vi "Tegam4040 -- Test Set-GetFilterMode.vi"() -> ()   [LabVIEW 2010]
panel:
  out "LP Filter Get":enum16{"No Filter", "100kHz", "1MHz"}(ring)
  in  "LP Filter Set":enum16{"No Filter", "100kHz", "1MHz"}(ring)
  out "error out":errorcluster
  in  "Tegam4040 Resource":refnum<visa-resource-name>
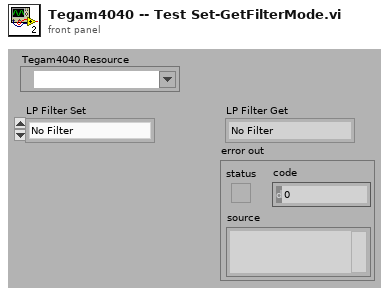
[diagram p1: front panel]
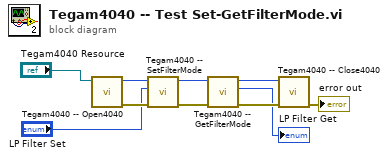
[diagram p0: block diagram]
diagram:
  n1 = call "Tegam4040 -- Open4040.vi"("VISA Resource In"="Tegam4040 Resource") -> ("error out"=w8:errorcluster, "Instrument Session Handle"=w9:u32)  [unwired: 9 in]
  n2 = call "Tegam4040 -- SetFilterMode.vi"("error in (no error)"=w8, "LP Filter"="LP Filter Set", "Instrument Session Handle In"=w9) -> ("error out"=w7:errorcluster, "Instrument Session Handle Out (dupl)"=w6:u32)  [unwired: 7 in]
  n3 = call "Tegam4040 -- GetFilterMode.vi"("error in (no error)"=w7, "Instrument Session Handle In"=w6) -> ("error out"=w5:errorcluster, "LP Filter"=→"LP Filter Get":enum16{"No Filter", "100kHz", "1MHz"}, "Instrument Session Handle Out (dupl)"=w4:u32)  [unwired: 7 in]
  n4 = call "Tegam4040 -- Close4040.vi"("error in (no error)"=w5, "Instrument Session Handle"=w4) -> ("error out"=→"error out":errorcluster)  [unwired: 9 in]
